vi "Laser Control.vi"(7 "Calling VI Ref":refnum<vi>) -> ()   [LabVIEW 2016]
uses:
  Laser Control Type Defs/Laser Control Control.ctl
  Hardware Configuration/Hardware Configuration Controls/Device Type.ctl
  <vilib>/Utility/miscctls.llb/LVPointTypeDef.ctl
  Device Library/Lasers/Laser Controls/Laser Actions.ctl
  Device Manager/Common Device Queue/Common Device Controls/Common Device Actions.ctl
  <vilib>/regexp/Match Regular Expression.xnode
panel:
  in  "Laser 05":T1={"Wavelength (nm)"=0, "Connect Text"="", "Connection"=TRUE, "Laser Status"="", "Emission"=TRUE, "Power (mW)"=0.0, "Settings"=TRUE}
  in  "Laser 04":T1={"Wavelength (nm)"=0, "Connect Text"="", "Connection"=TRUE, "Laser Status"="", "Emission"=TRUE, "Power (mW)"=0.0, "Settings"=TRUE}
  in  "Laser 03":T1={"Wavelength (nm)"=0, "Connect Text"="", "Connection"=TRUE, "Laser Status"="", "Emission"=TRUE, "Power (mW)"=0.0, "Settings"=TRUE}
  in  "Laser 02":T1={"Wavelength (nm)"=0, "Connect Text"="", "Connection"=TRUE, "Laser Status"="", "Emission"=TRUE, "Power (mW)"=0.0, "Settings"=TRUE}
  in  "Laser 01":T1={"Wavelength (nm)"=0, "Connect Text"="", "Connection"=TRUE, "Laser Status"="", "Emission"=TRUE, "Power (mW)"=0.0, "Settings"=TRUE}
  in  "Quit":bool
  # "Status:"
  # "Status:"
  # "Status:"
  # "Status:"
  # "Status:"
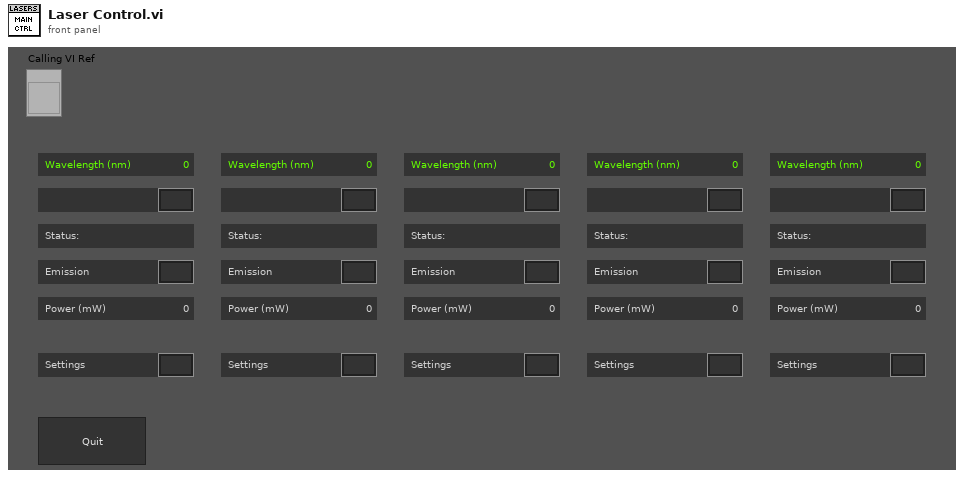
[diagram p1: front panel]
types:
  T1 = typedef "Laser Control Control.ctl" = cluster{"Wavelength (nm)":u16, "Connect Text":string, "Connection":bool, "Laser Status":string, "Emission":bool, "Power (mW)":dbl, "Settings":bool}
  T2 = enum16{"Always On", "Always Off", "Off While Running"}
  T3 = typedef "LVPointTypeDef.ctl" = cluster{"Horizontal":i16, "Vertical":i16}
  T4 = typedef "Device Type.ctl" = enum16{"AOTF", "Camera", "Deformable Mirror", "Laser", "Shutter", "Stage", "Waveform", "FPGA", "Email"}
  T5 = typedef "LVRectTypeDef.ctl" = cluster{"Left":i16, "Top":i16, "Right":i16, "Bottom":i16}
  T6 = typedef "LVBoundsTypeDef.ctl" = cluster{"Width":u32, "Height":u32}
  T7 = typedef "Laser Actions.ctl" = enum16{"Error Check", "Set On/Off", "Set Power", "Set Parameter", "Get Power", "Get Status", "Get Parameter", "Quit"}
  T8 = typedef "Common Device Actions.ctl" = enum16{"Specific Action", "Open Front Panel", "Close Front Panel", "Quit", "Quit All"}
  T9 = typedef "Laser Status.ctl" = enum16{"Warmup", "Ready", "Emission", "Tuning", "Error"}
  T10 = typedef "Device Function.ctl" = enum16{"Primary", "Secondary", "Overview", "Wide Field Drift Correction", "642 nm Excitation", "560 nm Excitation", "940 nm Excitation", "546 nm Excitation", "488 nm Excitation", "405 nm Excitation", "Objective Drift Correction", "4Pi Objective Lock", "Objective XY", "Objective Z", "Sample XY", "Sample Coarse Z", "Sample Z", "4Pi Lower", "4Pi Upper", "Mojo", "Adj Cavity", "Line Scanning", "Alert"}
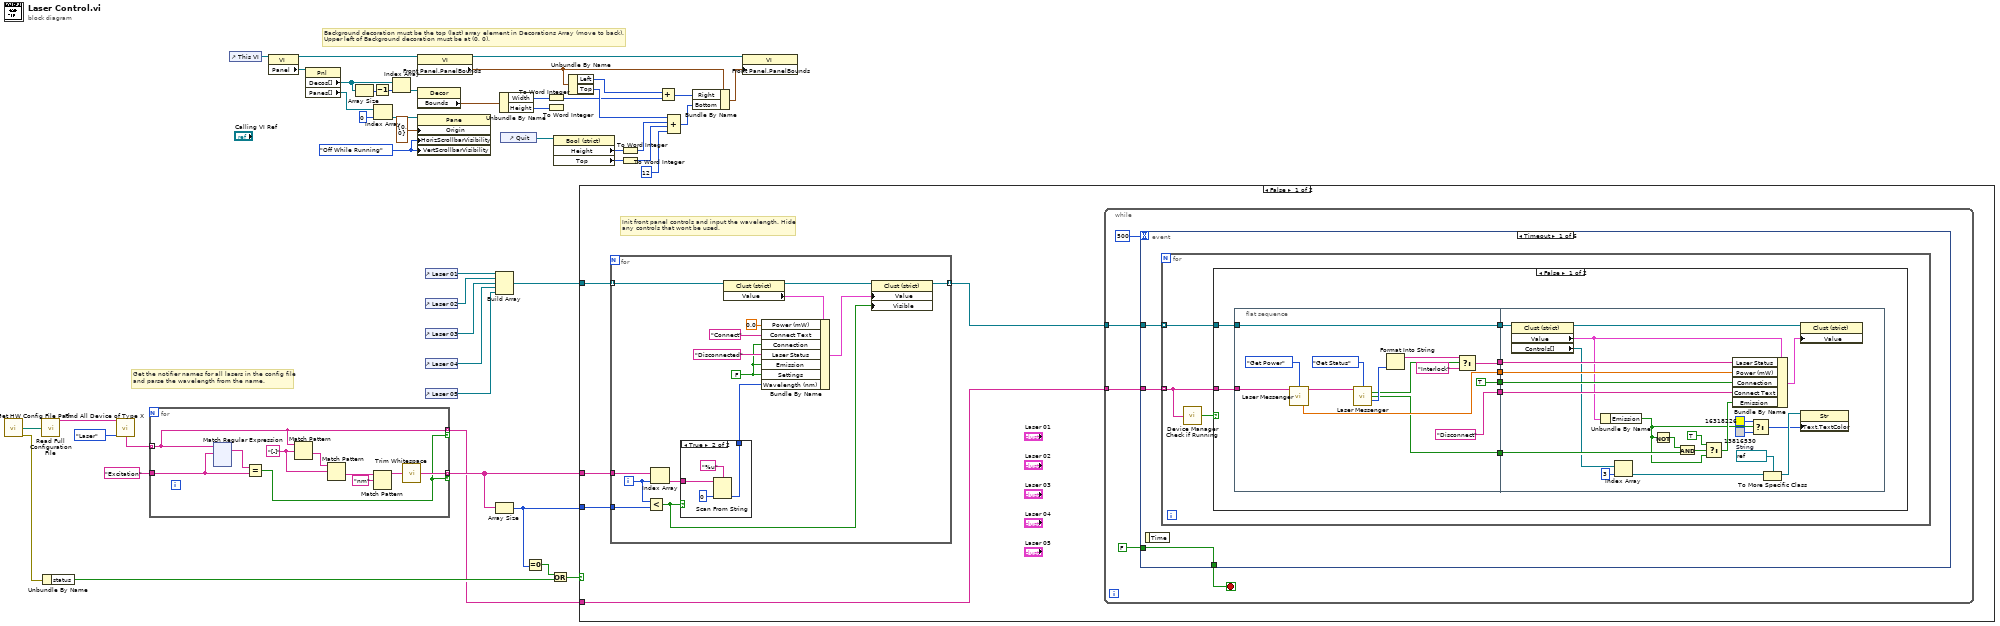
[diagram p0: block diagram]
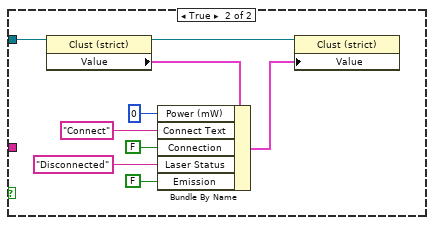
[diagram p2: hidden frame]
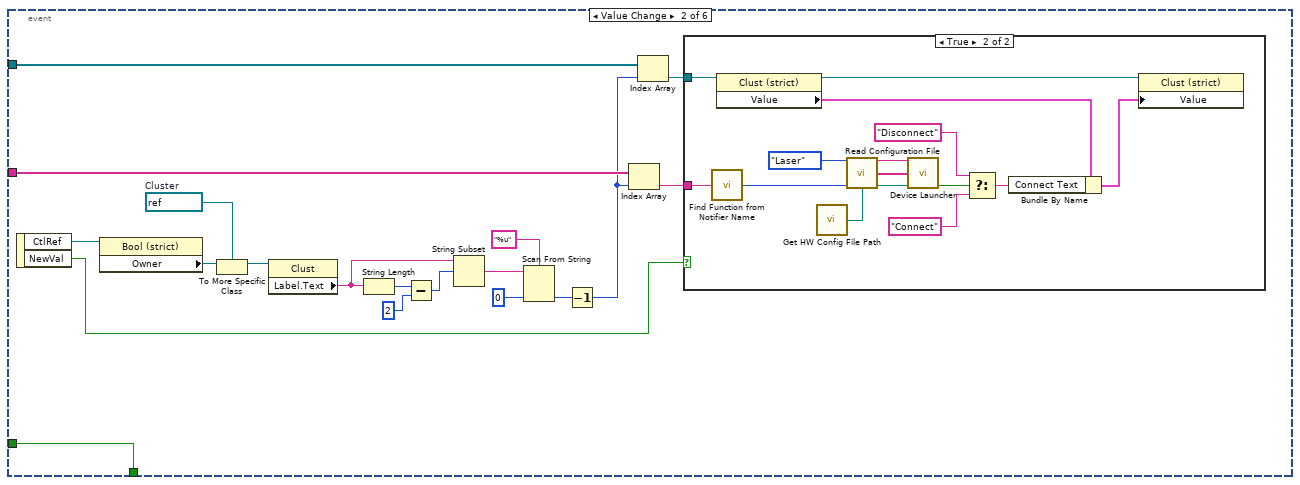
[diagram p3: hidden frame]
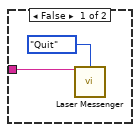
[diagram p4: hidden frame]
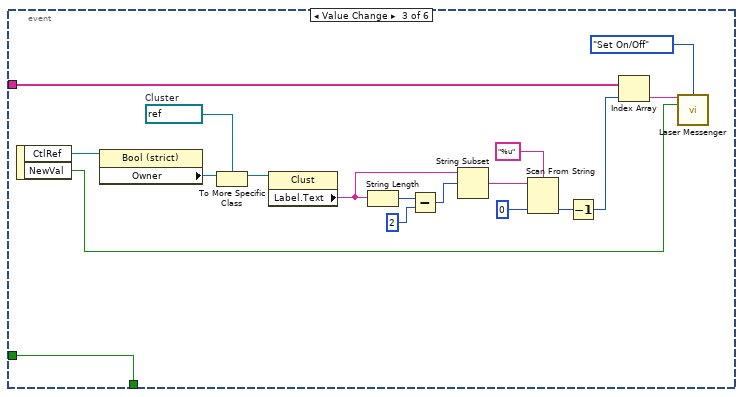
[diagram p5: hidden frame]
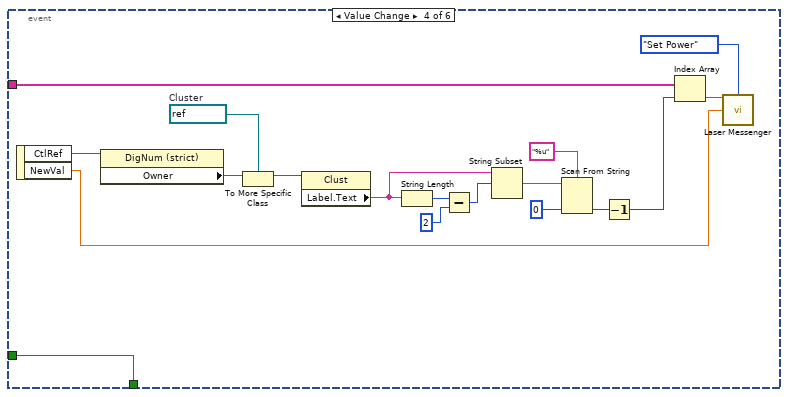
[diagram p6: hidden frame]
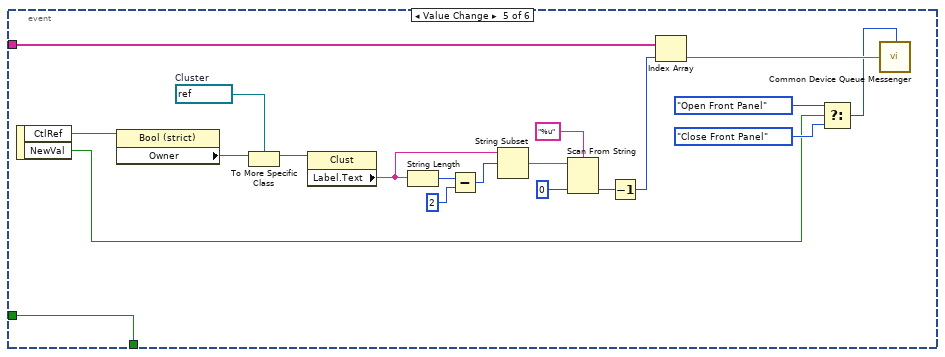
[diagram p7: hidden frame]
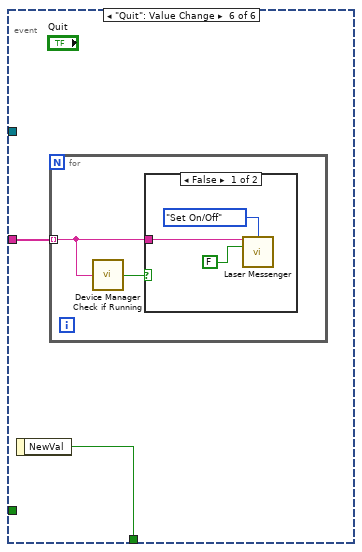
[diagram p8: hidden frame]
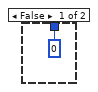
[diagram p10: hidden frame]
diagram:
  w27 = T2."Off While Running" ("Vertical Scrollbar Visibility")
  # "Get the notifier names for all lasers in the config file\nand parse the wavelength from the name."
  # "Background decoration must be the top (last) array element in Decorations Array (move to back).\nUpper left of Background decoration must be at (0, 0)."
  n1 = call "Get HW Config File Path.vi"() -> ("File Path"=w47:path, "Error"=w5:errorcluster)  [unwired: 14 in]
  n2 = call "Read Full Configuration File.vi"("Config File Path"=w47) -> ("Unique Notifier Names"=w46:string[])  [unwired: 11 in, 3 out]
  n3 = Unbundle By Name(w5) -> ("status"=w4:bool)
  n4 = call "Find All Device of Type X.vi"("Unique Notifier Names"=w46, "Device Type"=Device_Type."Laser") -> ("All Devices"=w10:string[])  [unwired: 12 in, 1 out]
  n5 = for {
    tunnel: w10 -> [w55] mode=indexing
    tunnel: [w55] -> w1 mode=indexing if=w48
    tunnel: "Excitation" -> [w56]
    tunnel: [w49] -> w3 mode=indexing if=w48
    w53 = "[-]" ("regular expression")
    n6 = xnode "Match Regular Expression"("input string"=w55, "regular expression"=w56) -> ("whole match"=w57:string)  [unwired: 4 in, 4 out]
    n7 = Equal?(x=w57, y=w56) -> (x = y?=w48:bool)
    n8 = Match Pattern(string=w55, regular expression=w53) -> (after substring=w54:string)  [unwired: 1 in, 3 out]
    n9 = Match Pattern(string=w54, regular expression=w53) -> (after substring=w52:string)  [unwired: 1 in, 3 out]
    n10 = Match Pattern(string=w52, regular expression="nm") -> (before substring=w50:string)  [unwired: 1 in, 3 out]
    n11 = call <vilib>:"Trim Whitespace.vi"("string"=w50) -> ("trimmed string"=w49:string)  [unwired: 1 in]
  }
  n12 = control-ref of="This VI"() -> (w19:refnum<vi>)
  n13 = property class="VI"(reference=w19) -> (reference out=w28:refnum<vi>, "Panel"=w20:refnum<vi>)  [unwired: 1 in, 1 out]
  n14 = property class="Pnl"(reference=w20) -> ("Decos[]"=w18:refnum<vi>[], "Panes[]"=w24:refnum<vi>[])  [unwired: 1 in, 2 out]
  n15 = Array Size(array=w18) -> (size(s)=w16:i32)
  n16 = Decrement(x=w16) -> (x-1=w17:i32)
  n17 = Index Array(array=w24, index=0) -> (element=w23:refnum<vi>)
  n18 = Index Array(array=w18, index=w17) -> (element=w26:refnum<vi>)
  n19 = property class="VI"(reference=w28) -> (reference out=w30:refnum<vi>, "Front Panel.PanelBounds"=w31:T5)  [unwired: 1 in, 1 out]
  n20 = property class="Decor"(reference=w26) -> ("Bounds"=w29:T6)  [unwired: 1 in, 2 out]
  n21 = property class="Pane"(reference=w23, "Origin"=T3 {"Horizontal"=0, "Vertical"=0}, "HorizScrollbarVisibility"=w27, "VertScrollbarVisibility"=w27) -> ()  [unwired: 1 in, 2 out]
  n22 = control-ref of="Laser 01"() -> (w15:refnum<vi>)
  n23 = control-ref of="Laser 02"() -> (w11:refnum<vi>)
  n24 = control-ref of="Laser 03"() -> (w12:refnum<vi>)
  n25 = control-ref of="Laser 04"() -> (w13:refnum<vi>)
  n26 = control-ref of="Laser 05"() -> (w14:refnum<vi>)
  n27 = Array Size(array=w3) -> (size(s)=w7:i32)
  n28 = Build Array(w15, w11, w12, w13, w14) -> (w8:refnum<vi>[])
  n29 = Unbundle By Name(w29) -> ("Width"=w34:u32, "Height"=w37:u32)
  n30 = control-ref of="Quit"() -> (w21:refnum<vi>)
  n31 = Equal To 0?(x=w7) -> (x = 0?=w6:bool)
  n32 = To Word Integer(number=w34) -> (16bit integer=w36:i16)
  n33 = To Word Integer(number=w37) -> ()  [unwired: 1 out]
  n34 = Or(x=w6, y=w4) -> (x .or. y?=w2:bool)
  n35 = property class="Bool (strict)"(reference=w21) -> ("Height"=w39:u32, "Top"=w40:i32)  [unwired: 1 in, 2 out]
  n36 = Unbundle By Name(w31) -> ("Left"=w33:i16, "Top"=w44:i16)
  n37 = case shown="False" w2 {
    tunnel: w8 -> [w176 _]
    tunnel: w7 -> [w175 _]
    tunnel: w3 -> [w174 _]
    tunnel: w1 -> [w172 _]
    frame False {
      # "Init front panel controls and input the wavelength. Hide\nany controls that wont be used."
      n38 = for {
        tunnel: w176 -> [w354] mode=indexing
        tunnel: w174 -> [w346]
        tunnel: [w347] -> w173 mode=indexing
        tunnel: w175 -> [w344]
        i -> [w345]
        w340 = FALSE ("Settings")
        n39 = Less?(x=w345, y=w344) -> (x < y?=w342:bool)
        n40 = Index Array(array=w346, index=w345) -> (element=w343:string)
        n41 = case shown="True" w342 {
          tunnel: [u16 0 ("default value 1") w357] -> w341
          tunnel: w343 -> [_ w356]
          frame False {
          }
          frame True {
            n42 = Scan From String(format string="%u", input string=w356, default 1=u16 0 ("default value 1")) -> (output 1=w357:u16)  [unwired: 2 in, 3 out]
          }
        }
        n43 = property class="Clust (strict)"(reference=w354) -> (reference out=w351:refnum<vi>, "Value"=w353:T1)  [unwired: 1 in, 1 out]
        n44 = Bundle By Name(cluster=w353, "Power (mW)"=0.0, "Connect Text"="Connect", "Connection"=w340, "Laser Status"="Disconnected", "Emission"=w340, "Settings"=w340, "Wavelength (nm)"=w341) -> (w350:T1)
        n45 = property class="Clust (strict)"(reference=w351, "Value"=w350, "Visible"=w342) -> (reference out=w347:refnum<vi>)  [unwired: 1 in, 1 out]
      }
      n46 = while {
        tunnel: w172 -> [w180]
        tunnel: w173 -> [w179]
        stop <- w178 stop-if-true
        n47 = event shown="[0] Timeout" {
          selector: _ -> [_ _ _ _ _ _]
          dyn-events: _ -> [_ _ _ _ _ _]
          timeout: 500 -> [_ _ _ _ _ _]
          tunnel: w180 -> [w184 w252 w286 w304 w317 w333]
          tunnel: w179 -> [w183 w250 _ _ _ _]
          tunnel: [w182 w259 w294 w312 w332 w334] -> w178
          tunnel: FALSE -> [w182 w259 w294 w312 w332 _]
          event Timeout {
            n48 = event-data() -> ()  [unwired: 1 in, 1 out]
            n49 = for {
              tunnel: w184 -> [w186] mode=indexing
              tunnel: w183 -> [w187] mode=indexing
              n50 = call "Device Manager Check if Running.vi"("Notifier Name"=w186) -> ("Running?"=w185:bool)  [unwired: 14 in]
              n51 = case shown="False" w185 {
                tunnel: w187 -> [w189 w240]
                tunnel: w186 -> [w195 _]
                frame False {
                  n52 = flat-sequence {
                    tunnel: w195 -> [w201]
                    tunnel: [w204] -> w194
                    tunnel: [w200] -> w193
                    tunnel: ["Disconnect" ("Connect Text")] -> w192
                    tunnel: [TRUE ("Connection")] -> w191
                    tunnel: [w197] -> w190
                    tunnel: w189 -> [w197]
                    tunnel: [w196] -> w188
                    tunnel: w194 -> [w229]
                    tunnel: w193 -> [w228]
                    tunnel: w192 -> [w226]
                    tunnel: w191 -> [w227]
                    tunnel: w190 -> [w225]
                    tunnel: w188 -> [w223]
                    frame #0 {
                      n53 = call "Laser Messenger.vi"("Notifier Name"=w201, "Action"=Laser_Actions."Get Power") -> ("Notifier Name Dup"=w203:string, "Power (mW)"=w200:dbl)  [unwired: 8 in, 4 out]
                      n54 = call "Laser Messenger.vi"("Notifier Name"=w203, "Action"=Laser_Actions."Get Status") -> ("Enabled (Interlock)?"=w207:bool, "Light Emission?"=w196:bool, "Laser Status"=w208:T9)  [unwired: 8 in, 3 out]
                      n55 = Format Into String(w208) -> (resulting string=w206:string)  [unwired: 3 in, 1 out]
                      n56 = Select(t=w206, s=w207, f="Interlock") -> (s? t:f=w204:string)
                    }
                    frame #1 {
                      w216 = refnum<vi> refnum  # String
                      n57 = property class="Clust (strict)"(reference=w225) -> (reference out=w231:refnum<vi>, "Value"=w224:T1, "Controls[]"=w218:refnum<vi>[])  [unwired: 1 in, 1 out]
                      n58 = Unbundle By Name(w224) -> ("Emission"=w213:bool)
                      n59 = Index Array(array=w218, index=3) -> (element=w210:refnum<vi>)
                      n60 = Not(x=w213) -> (.not. x?=w222:bool)
                      n61 = And(x=w222, y=w223) -> (x .and. y?=w221:bool)
                      n62 = Select(t=TRUE, s=w221, f=w213) -> (s? t:f=w219:bool)
                      n63 = Bundle By Name(cluster=w224, "Laser Status"=w229, "Power (mW)"=w228, "Connection"=w227, "Connect Text"=w226, "Emission"=w219) -> (w230:T1)
                      n64 = Select(t=u32 16318226 ("Color Box"), s=w213, f=u32 13816530) -> (s? t:f=w211:u32)
                      n65 = To More Specific Class(target class=w216, reference=w210) -> (specific class reference=w215:refnum<vi>)  [unwired: 1 in, 1 out]
                      n66 = property class="Str"(reference=w215, "Text.TextColor"=w211) -> ()  [unwired: 1 in, 2 out]
                      n67 = property class="Clust (strict)"(reference=w231, "Value"=w230) -> ()  [unwired: 1 in, 2 out]
                    }
                  }
                }
                frame True {
                  n68 = property class="Clust (strict)"(reference=w240) -> (reference out=w233:refnum<vi>, "Value"=w234:T1)  [unwired: 1 in, 1 out]
                  n69 = Bundle By Name(cluster=w234, "Power (mW)"=u16 0, "Connect Text"="Connect", "Connection"=FALSE, "Laser Status"="Disconnected", "Emission"=FALSE) -> (w232:T1)
                  n70 = property class="Clust (strict)"(reference=w233, "Value"=w232) -> ()  [unwired: 1 in, 2 out]
                }
              }
            }
          }
          event Value Change {
            w246 = refnum<vi> refnum  # Cluster
            n71 = event-data() -> ("CtlRef"=w244:refnum<vi>, "NewVal"=w241:bool)  [unwired: 1 in]
            n72 = property class="Bool (strict)"(reference=w244) -> ("Owner"=w245:refnum<vi>)  [unwired: 1 in, 2 out]
            n73 = To More Specific Class(target class=w246, reference=w245) -> (specific class reference=w247:refnum<vi>)  [unwired: 1 in, 1 out]
            n74 = property class="Clust"(reference=w247) -> ("Label.Text"=w243:string)  [unwired: 1 in, 2 out]
            n75 = String Length(string=w243) -> (length=w258:i32)
            n76 = Subtract(x=w258, y=2) -> (x-y=w256:i32)
            n77 = String Subset(string=w243, offset (0)=w256) -> (substring=w253:string)  [unwired: 1 in]
            n78 = Scan From String(format string="%u", input string=w253, default 1=0) -> (output 1=w249:i32)  [unwired: 2 in, 3 out]
            n79 = Decrement(x=w249) -> (x-1=w242:i32)
            n80 = Index Array(array=w252, index=w242) -> (element=w251:string)
            n81 = Index Array(array=w250, index=w242) -> (element=w248:refnum<vi>)
            n82 = case shown="True" w241 {
              tunnel: w251 -> [w260 w271]
              tunnel: w248 -> [_ w269]
              frame False {
                n83 = call "Laser Messenger.vi"("Notifier Name"=w260, "Action"=Laser_Actions."Quit") -> ()  [unwired: 8 in, 6 out]
              }
              frame True {
                n84 = call "Find Function from Notifier Name.vi"("Unique Notifier Name"=w271) -> ("Function"=w270:T10)  [unwired: 14 in]
                n85 = property class="Clust (strict)"(reference=w269) -> (reference out=w263:refnum<vi>, "Value"=w268:T1)  [unwired: 1 in, 1 out]
                n86 = call "Get HW Config File Path.vi"() -> ("File Path"=w275:path)  [unwired: 14 in, 1 out]
                n87 = call "Read Configuration File.vi"("Device Type"=Device_Type."Laser", "Device Function"=w270, "Config File Path"=w275) -> ("Unique Notifier Name"=w274:string, "Device Ports/IDs/Channels"=w272:string[], "Device Engine Path"=w273:path)  [unwired: 9 in, 1 out]
                n88 = call "Device Launcher.vi"("Notifier Name"=w274, "Device Ports/IDs/Channels"=w272, "Device Engine Path"=w273) -> ("Running?"=w267:bool)  [unwired: 11 in, 1 out]
                n89 = Select(t="Disconnect", s=w267, f="Connect") -> (s? t:f=w264:string)
                n90 = Bundle By Name(cluster=w268, "Connect Text"=w264) -> (w262:T1)
                n91 = property class="Clust (strict)"(reference=w263, "Value"=w262) -> ()  [unwired: 1 in, 2 out]
              }
            }
          }
          event Value Change {
            w282 = refnum<vi> refnum  # Cluster
            n92 = event-data() -> ("CtlRef"=w280:refnum<vi>, "NewVal"=w278:bool)  [unwired: 1 in]
            n93 = property class="Bool (strict)"(reference=w280) -> ("Owner"=w281:refnum<vi>)  [unwired: 1 in, 2 out]
            n94 = To More Specific Class(target class=w282, reference=w281) -> (specific class reference=w283:refnum<vi>)  [unwired: 1 in, 1 out]
            n95 = property class="Clust"(reference=w283) -> ("Label.Text"=w279:string)  [unwired: 1 in, 2 out]
            n96 = String Length(string=w279) -> (length=w293:i32)
            n97 = Subtract(x=w293, y=2) -> (x-y=w291:i32)
            n98 = String Subset(string=w279, offset (0)=w291) -> (substring=w288:string)  [unwired: 1 in]
            n99 = Scan From String(format string="%u", input string=w288, default 1=0) -> (output 1=w287:i32)  [unwired: 2 in, 3 out]
            n100 = Decrement(x=w287) -> (x-1=w277:i32)
            n101 = Index Array(array=w286, index=w277) -> (element=w285:string)
            n102 = call "Laser Messenger.vi"("Notifier Name"=w285, "Action"=Laser_Actions."Set On/Off", "Emission On/Off"=w278) -> ()  [unwired: 7 in, 6 out]
          }
          event Value Change {
            w299 = refnum<vi> refnum  # Cluster
            n103 = event-data() -> ("CtlRef"=w297:refnum<vi>, "NewVal"=w301:dbl)  [unwired: 1 in]
            n104 = property class="DigNum (strict)"(reference=w297) -> ("Owner"=w298:refnum<vi>)  [unwired: 1 in, 2 out]
            n105 = To More Specific Class(target class=w299, reference=w298) -> (specific class reference=w300:refnum<vi>)  [unwired: 1 in, 1 out]
            n106 = property class="Clust"(reference=w300) -> ("Label.Text"=w296:string)  [unwired: 1 in, 2 out]
            n107 = String Length(string=w296) -> (length=w311:i32)
            n108 = Subtract(x=w311, y=2) -> (x-y=w309:i32)
            n109 = String Subset(string=w296, offset (0)=w309) -> (substring=w306:string)  [unwired: 1 in]
            n110 = Scan From String(format string="%u", input string=w306, default 1=0) -> (output 1=w305:i32)  [unwired: 2 in, 3 out]
            n111 = Decrement(x=w305) -> (x-1=w295:i32)
            n112 = Index Array(array=w304, index=w295) -> (element=w303:string)
            n113 = call "Laser Messenger.vi"("Notifier Name"=w303, "Action"=Laser_Actions."Set Power", "Power (mW)"=w301) -> ()  [unwired: 7 in, 6 out]
          }
          event Value Change {
            w321 = refnum<vi> refnum  # Cluster
            n114 = event-data() -> ("CtlRef"=w318:refnum<vi>, "NewVal"=w314:bool)  [unwired: 1 in]
            n115 = property class="Bool (strict)"(reference=w318) -> ("Owner"=w320:refnum<vi>)  [unwired: 1 in, 2 out]
            n116 = To More Specific Class(target class=w321, reference=w320) -> (specific class reference=w322:refnum<vi>)  [unwired: 1 in, 1 out]
            n117 = property class="Clust"(reference=w322) -> ("Label.Text"=w319:string)  [unwired: 1 in, 2 out]
            n118 = String Length(string=w319) -> (length=w329:i32)
            n119 = Subtract(x=w329, y=2) -> (x-y=w327:i32)
            n120 = String Subset(string=w319, offset (0)=w327) -> (substring=w324:string)  [unwired: 1 in]
            n121 = Scan From String(format string="%u", input string=w324, default 1=0) -> (output 1=w323:i32)  [unwired: 2 in, 3 out]
            n122 = Decrement(x=w323) -> (x-1=w316:i32)
            n123 = Index Array(array=w317, index=w316) -> (element=w315:string)
            n124 = Select(t=Common_Device_Actions."Open Front Panel" ("Common Actions"), s=w314, f=Common_Device_Actions."Close Front Panel" ("Common Actions")) -> (s? t:f=w313:T8)
            n125 = call "Common Device Queue Messenger.vi"("Common Action"=w313, "Notifier Name"=w315) -> ()  [unwired: 13 in, 1 out]
          }
          event "Quit": Value Change {
            n126 = event-data() -> ("NewVal"=w334:bool)  [unwired: 1 in]
            n127 = for {
              tunnel: w333 -> [w336] mode=indexing
              n128 = call "Device Manager Check if Running.vi"("Notifier Name"=w336) -> ("Running?"=w335:bool)  [unwired: 14 in]
              n129 = case shown="False" w335 {
                tunnel: w336 -> [w337 _]
                frame False {
                  n130 = call "Laser Messenger.vi"("Notifier Name"=w337, "Action"=Laser_Actions."Set On/Off", "Emission On/Off"=FALSE) -> ()  [unwired: 7 in, 6 out]
                }
                frame True {
                }
              }
            }
          }
        }
      }
    }
    frame True {
    }
  }
  n131 = To Word Integer(number=w39) -> (16bit integer=w42:i16)
  n132 = To Word Integer(number=w40) -> (16bit integer=w43:i16)
  n133 = Add(x=w33, y=w36) -> (x+y=w35:i16)
  n134 = Compound Arithmetic op=ADD(w44, w42, w43, i16 12 ("y")) -> (w38:i16)
  n135 = Bundle By Name(cluster=w31, "Right"=w35, "Bottom"=w38) -> (w32:T5)
  n136 = property class="VI"(reference=w30, "Front Panel.PanelBounds"=w32) -> ()  [unwired: 1 in, 2 out]
